vi "Read Global Locked.vi"(7 "Semaphore Timeout":i32=-1, 8 "error in (no error)":errorcluster, 11 "GrabberArms in":refnum<class "GrabberArms.lvclass">) -> (0 "error out":errorcluster, 1 "Semaphore Timed Out":bool, 2 "Global":refnum<class "System.lvclass">, 3 "GrabberArms out":refnum<class "GrabberArms.lvclass">)   [LabVIEW 2013, in "GrabberArms.lvclass"]
uses:
  GrabberArms.lvclass
  System/System.lvclass
  Robot Global Data.vi
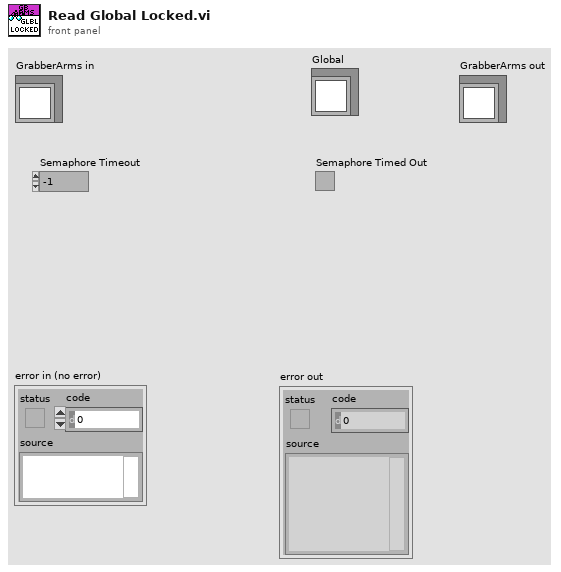
[diagram p1: front panel]
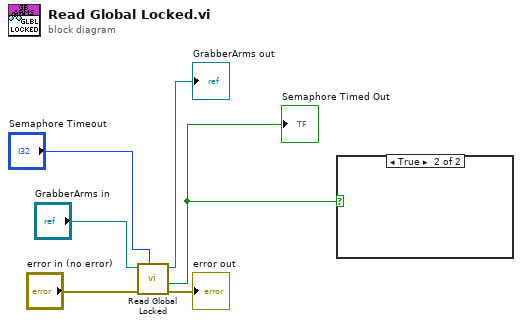
[diagram p0: block diagram]
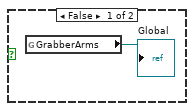
[diagram p2: hidden frame]
diagram:
  n1 = call-parent "Read Global Locked.vi"("Semaphore Timeout"="Semaphore Timeout", "error in (no error)"="error in (no error)", "System in"="GrabberArms in") -> ("error out"=→"error out":errorcluster, "Semaphore Timed Out"=w1:bool, "System out"=→"GrabberArms out":refnum<class "GrabberArms.lvclass">)  [unwired: 5 in, 1 out]
  "Semaphore Timed Out" <- w1
  n2 = case shown="True" w1 {
    frame False {
      n3 = global read "Robot Global Data.vi" "GrabberArms"() -> (→"Global":refnum<class "GrabberArms.lvclass">)
    }
    frame True {
    }
  }
